vi "Point_DoesTagExist_Internal.vi"(0 "Map":variant, 5 "Tag":string, 11 "Error In":errorcluster) -> (4 "Map Out":variant, 6 "Tag Out":string, 8 "Tag Exists":bool, 10 "Point":T2, 14 "Datatype":T1, 15 "Error Out":errorcluster)   [LabVIEW 2017, in "PointValueMap.lvlib"]
uses:
  <vilib>/addons/PointValueMap/PointValueMap.lvlib
  <vilib>/addons/PointValueMap/controls/Point.ctl
  <vilib>/addons/PointValueMap/controls/DataTypes.ctl
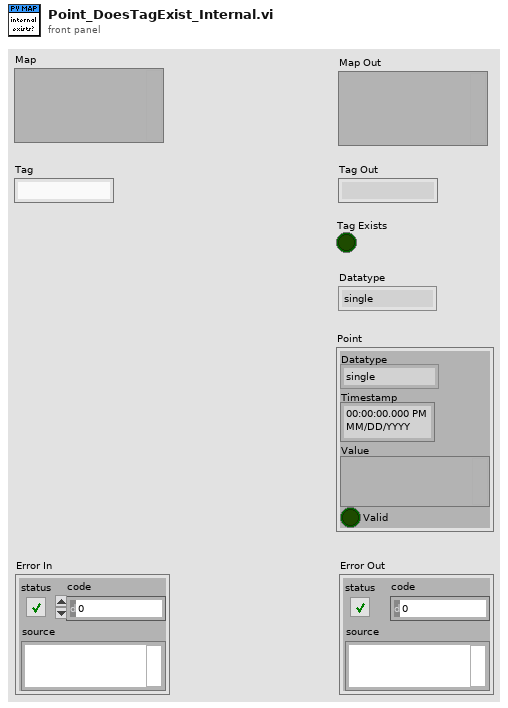
[diagram p1: front panel]
types:
  T1 = typedef "PointValueMap.lvlib/DataTypes.ctl" = enum16{"single", "double", "i32", "string", "variant"}
  T2 = typedef "PointValueMap.lvlib/Point.ctl" = cluster{"Datatype":T1, "Timestamp":timestamp, "Value":variant, "Valid":bool}
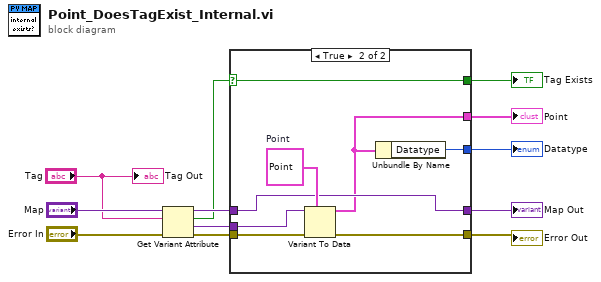
[diagram p0: block diagram]
diagram:
  n1 = Get Variant Attribute(Variant="Map", name="Tag", error in="Error In") -> (duplicate Variant=w11:variant, found=w7:bool, value=w3:variant, error out=w9:errorcluster)  [unwired: 1 in]
  n2 = case shown="True" w7 {
    selector: w7 -> [w15 w23]
    tunnel: w11 -> [w14 w19]
    tunnel: w9 -> [w13 w22]
    tunnel: [w14 w19] -> w8
    tunnel: [w15 w23] -> w6
    tunnel: [w13 w18] -> w4
    tunnel: w3 -> [_ w21]
    tunnel: [_ w17] -> w2
    tunnel: [_ w16] -> w1
    frame False {
    }
    frame True {
      w20 = T2 {"Datatype"=enum."single", "Timestamp"=timestamp(0 s since 1904-01-01), "Value"=variant, "Valid"=FALSE}  # Point
      n3 = Variant To Data(error in=w22, type=w20, Variant=w21) -> (data=w17:T2, error out=w18:errorcluster)
      n4 = Unbundle By Name(w17) -> ("Datatype"=w16:T1)
    }
  }
  "Tag Exists" <- w6
  "Map Out" <- w8
  "Error Out" <- w4
  "Point" <- w2
  "Datatype" <- w1
  "Tag Out" <- "Tag"
